vi "FTW-ProjectManager-RegisterApplicationShutdownEvent.vi"(0 "Project Manager":refnum<class "FTW-ProjectManager.lvclass">, 11 "error in":errorcluster) -> (4 "Project Manager out":refnum<class "FTW-ProjectManager.lvclass">, 6 "Application Shutdown Event":refnum<event-registration>, 15 "error out":errorcluster)   [LabVIEW 2012, in "FTW-ProjectManager.lvclass"]
uses:
  FTW-ProjectManager.lvclass
panel:
  # "Inputs"
  # "Outputs"
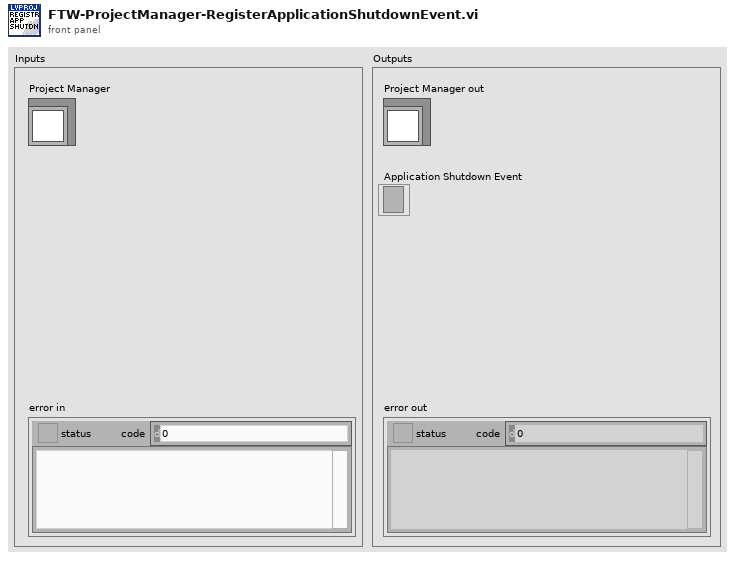
[diagram p1: front panel]
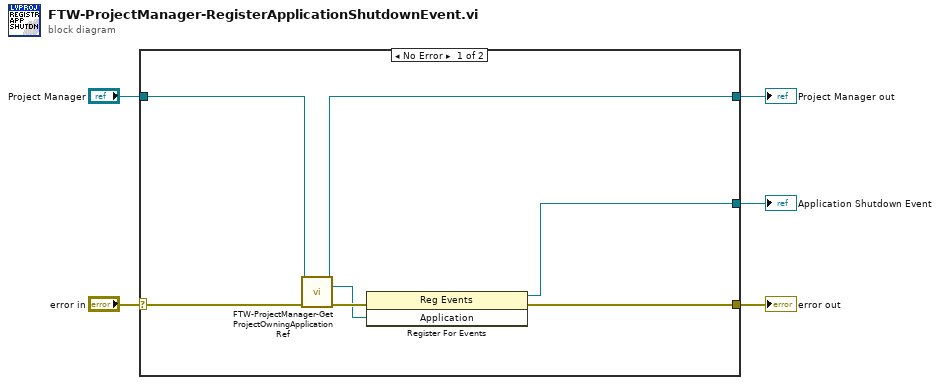
[diagram p0: block diagram]
diagram:
  n1 = case shown="No Error" "error in" {
    selector: "error in" -> [w8 w14]
    tunnel: [w12 w14] -> w5
    tunnel: [w9 w13] -> w3
    tunnel: "Project Manager" -> [w10 w13]
    tunnel: [w11 _] -> w1
    frame No Error {
      n2 = call "FTW-ProjectManager-GetProjectOwningApplicationRef.vi"("Project Manager"=w10, "error in"=w8) -> ("Project Manager out"=w9:refnum<class "FTW-ProjectManager.lvclass">, "Application"=w6:refnum<vi>, "error out"=w7:errorcluster)  [unwired: 9 in, 2 out]
      n3 = register-events(error in=w7, w6) -> (reference out=w11:refnum<event-registration>, error out=w12:errorcluster)  [unwired: 1 in]
    }
    frame Error {
    }
  }
  "error out" <- w5
  "Project Manager out" <- w3
  "Application Shutdown Event" <- w1
